vi "Check info str.vi"(8 "error in (no error)":errorcluster, 10 "Data in":string, 11 "Motor info":T1={"Motor positions"=[0.0, 0.0], "Sensor value"=0.0, "End-stop state"=[FALSE, FALSE], "°/step"=[], "Motor params"={"Action"=2, "Direction motor 1"=1, "Direction motor 2"=1, "Steps motor 1"=100, "Steps motor 2"=100, "Step style motor 1"=1, "Step style motor 2"=1}, "Moving?"=FALSE, "Home?"=FALSE, "Connected?"=FALSE, "Manual zero?"=FALSE} {"Motor params"."Step style motor 2" items=["", "Single", "Double", "Interleave", "Microstep"]; "Motor params"."Step style motor 1" items=["", "Single", "Double", "Interleave", "Microstep"]; "Motor params"."Direction motor 2" items=["", "Forward", "Backward"]; "Motor params"."Direction motor 1" items=["", "Forward", "Backward"]; "Motor params"."Action" items=["", "Initialize", "Move"]; "°/step" format="%#_13g"}) -> (0 "error out":errorcluster, 1 "Home?":bool, 2 "End?":bool, 3 "Motor info out":T1={"Motor positions"=[0.0, 0.0], "Sensor value"=0.0, "End-stop state"=[FALSE, FALSE], "°/step"=[], "Motor params"={"Action"=2, "Direction motor 1"=1, "Direction motor 2"=1, "Steps motor 1"=100, "Steps motor 2"=100, "Step style motor 1"=1, "Step style motor 2"=1}, "Moving?"=FALSE, "Home?"=FALSE, "Connected?"=FALSE, "Manual zero?"=FALSE} {"Motor params"."Step style motor 2" items=["", "Single", "Double", "Interleave", "Microstep"]; "Motor params"."Step style motor 1" items=["", "Single", "Double", "Interleave", "Microstep"]; "Motor params"."Direction motor 2" items=["", "Forward", "Backward"]; "Motor params"."Direction motor 1" items=["", "Forward", "Backward"]; "Motor params"."Action" items=["", "Initialize", "Move"]; "°/step" format="%#_13g"})   [LabVIEW 2020, in "Control de MaP.lvlib"]
uses:
  Control de MaP.lvlib
  Controls/Motor info.ctl
  Controls/Move motor parameters--cluster.ctl
  Controls/Motor direction.ctl
  Controls/Step style.ctl
  Arduino-Adafruit stepper/Arduino-Adafruit stepper.lvlib
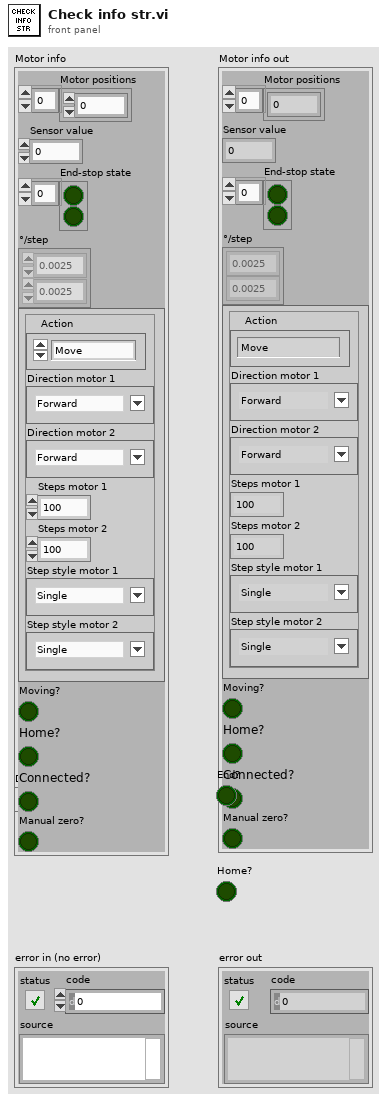
[diagram p1: front panel]
types:
  T1 = typedef "Arduino-Adafruit stepper.lvlib/Motor info.ctl" = cluster{"Motor positions":dbl[], "Sensor value":dbl, "End-stop state":bool[], "°/step":dbl[], "Motor params":T2, "Moving?":bool, "Home?":bool, "Connected?":bool, "Manual zero?":bool}
  T2 = typedef "Arduino-Adafruit stepper.lvlib/Move motor parameters--cluster.ctl" = cluster{"Action":u8, "Direction motor 1":T3, "Direction motor 2":T3, "Steps motor 1":u16, "Steps motor 2":u16, "Step style motor 1":T4, "Step style motor 2":T4}
  T3 = typedef "Arduino-Adafruit stepper.lvlib/Motor direction.ctl" = u8
  T4 = typedef "Arduino-Adafruit stepper.lvlib/Step style.ctl" = u8
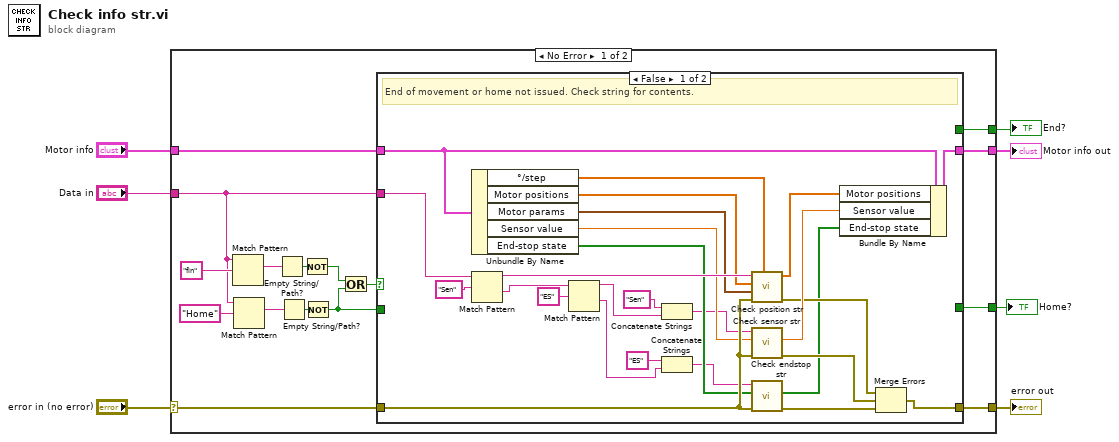
[diagram p0: block diagram]
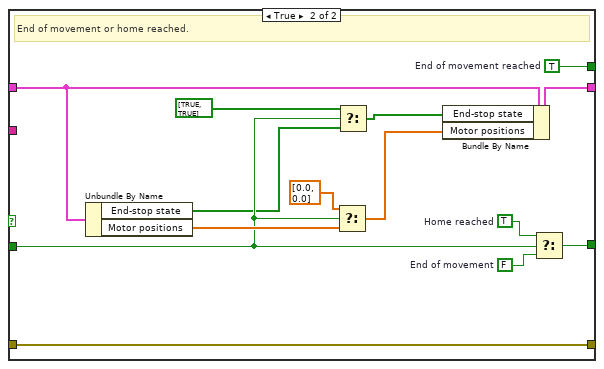
[diagram p2: hidden frame]
diagram:
  n1 = case shown="No Error" "error in (no error)" {
    selector: "error in (no error)" -> [w22 w65]
    tunnel: "Data in" -> [w15 _]
    tunnel: [w21 w65] -> w5
    tunnel: "Motor info" -> [w23 w64]
    tunnel: [w20 w64] -> w3
    tunnel: [w17 _] -> w2
    tunnel: [w11 _] -> w1
    frame No Error {
      n2 = Match Pattern(string=w15, regular expression="fin") -> (match substring=w18:string)  [unwired: 1 in, 3 out]
      n3 = Match Pattern(string=w15, regular expression="Home") -> (match substring=w14:string)  [unwired: 1 in, 3 out]
      n4 = Empty String/Path?(string/path=w18) -> (empty?=w13:bool)
      n5 = Empty String/Path?(string/path=w14) -> (empty?=w10:bool)
      n6 = Not(x=w13) -> (.not. x?=w9:bool)
      n7 = Not(x=w10) -> (.not. x?=w8:bool)
      n8 = Or(x=w9, y=w8) -> (x .or. y?=w12:bool)
      n9 = case shown="False" w12 {
        tunnel: w15 -> [w46 _]
        tunnel: w23 -> [w43 w58]
        tunnel: w22 -> [w40 w62]
        tunnel: [w36 w62] -> w21
        tunnel: [w34 w57] -> w20
        tunnel: [_ w63] -> w17
        tunnel: [_ w61] -> w11
        tunnel: w8 -> [_ w53]
        frame False {
          # "End of movement or home not issued. Check string for contents."
          n10 = Unbundle By Name(w43) -> ("°/step"=w35:dbl[], "Motor positions"=w44:dbl[], "Motor params"=w33:T2, "Sensor value"=w32:dbl, "End-stop state"=w31:bool[])
          n11 = Match Pattern(string=w46, regular expression="Sen") -> (before substring=w45:string, after substring=w48:string)  [unwired: 1 in, 2 out]
          n12 = Match Pattern(string=w48, regular expression="ES") -> (before substring=w30:string, after substring=w26:string)  [unwired: 1 in, 2 out]
          n13 = Concatenate Strings("Sen" ("string"), w30) -> (w28:string)
          n14 = Concatenate Strings("ES" ("string"), w26) -> (w25:string)
          n15 = call "Check position str.vi"("°/step"=w35, "error in (no error)"=w40, "Motor params"=w33, "Positions"=w44, "Recibo de Datos"=w45) -> ("error out"=w39:errorcluster, "Positions out"=w42:dbl[])  [unwired: 5 in]
          n16 = call "Check sensor str.vi"("error in (no error)"=w40, "Sensor value in"=w32, "string"=w28) -> ("error out"=w38:errorcluster, "Sensor value out"=w41:dbl)  [unwired: 6 in]
          n17 = call "Check endstop str.vi"("error in (no error)"=w40, "Ens-stop state in"=w31, "Data in"=w25) -> ("error out"=w37:errorcluster, "Ens-stop state out"=w24:bool[])  [unwired: 7 in]
          n18 = Bundle By Name(cluster=w43, "Motor positions"=w42, "Sensor value"=w41, "End-stop state"=w24) -> (w34:T1)
          n19 = Merge Errors(w39, w38, w37) -> (w36:errorcluster)
        }
        frame True {
          w59 = FALSE  # End of movement
          w60 = TRUE  # Home reached
          w63 = TRUE  # End of movement reached
          # "End of movement or home reached."
          n20 = Unbundle By Name(w58) -> ("End-stop state"=w52:bool[], "Motor positions"=w56:dbl[])
          n21 = Select(t=dbl[] [0.0, 0.0] ("Motor positions"), s=w53, f=w56) -> (s? t:f=w54:dbl[])
          n22 = Select(t=bool[] [TRUE, TRUE], s=w53, f=w52) -> (s? t:f=w50:bool[])
          n23 = Bundle By Name(cluster=w58, "End-stop state"=w50, "Motor positions"=w54) -> (w57:T1)
          n24 = Select(t=w60, s=w53, f=w59) -> (s? t:f=w61:bool)
        }
      }
    }
    frame Error {
    }
  }
  "error out" <- w5
  "Motor info out" <- w3
  "End?" <- w2
  "Home?" <- w1
